vi "play_FXP_AFMss_LinearDistEst_singleAxis.vi"() -> ()   [LabVIEW 2017]
uses:
  fpga_VIs/fpga_subVIs_ssxy/fixed-point-ss/typeDefs/FXPControlParams_distEst.ctl
  fpga_fp_interface_lib/fpga_interface_types/boolean_indicators.ctl
  <vilib>/Analysis/Matrix/Datatypes/RealMatrix.ctl
  <vilib>/userdefined/High Color/nirio_resource_hc.ctl
  <vilib>/Utility/error.llb/DialogType.ctl
  <vilib>/Analysis/Matrix/Numeric/Conversions/Matrix To Array - RM.vi
  <vilib>/Utility/file.llb/Read Delimited Spreadsheet (DBL).vi
  <vilib>/FPGAPlugInAG/cRIO-9082/niLvFpga_Open_cRIO-9082.vi
  <vilib>/rvi/interface/common/dynamic/niFpgaDynamicAddResources.vi
  <vilib>/FPGAPlugInAG/Dynamic/niLvFpga_Reset_Dynamic.vi
  <vilib>/rvi/interface/common/niFpgaWaitOnOcc.vi
  <vilib>/Utility/error.llb/Error Cluster From Error Code.vi
  <vilib>/rvi/errors/niLvFpgaAdjustHostInterfaceError.vi
  <vilib>/FPGAPlugInAG/Dynamic/niLvFpga_Run_Dynamic.vi
  <vilib>/RVI Host/nirviSupport.llb/nirviErrorClusterFromErrorCode.vi
  fpga_fp_interface_lib/write_FP_data_to_fpga.vi
  fpga_fp_interface_lib/acquire_FXP_18-5_FIFO_1.vi
  <vilib>/Utility/file.llb/Write To Spreadsheet File (DBL).vi
  <vilib>/Analysis/Matrix/Numeric/Conversions/Array To Matrix - RA2.vi
  <vilib>/FPGAPlugInAG/Dynamic/niLvFpga_Close_Dynamic.vi
  <vilib>/rvi/interface/nirviOpenFPGA/nirviOpenFPGA.xnode
  FPGA Bitfiles/afmimagingcontro_FPGATargetSPARTA_FXPAFMssLinearDi_nzyJCj76J+U.lvbitx
  <vilib>/rvi/interface/nirviMethod/nirviMethod.xnode
  <vilib>/rvi/interface/nirviReadWriteControl/nirviReadWriteControl.xnode
  <vilib>/rvi/interface/nirviCloseFPGA/nirviCloseFPGA.xnode
  <vilib>/rvi/errors/niLvFpgaMergeErrorWithErrorCode.vi
  <vilib>/rvi/interface/Simulation/niFpgaSimulationCallBeginRW.vi
  <vilib>/rvi/interface/nirviMethod/StockFPGA_InlinedMethodWaitForSingleIRQ.vi
  <vilib>/FPGAPlugInAG/Dynamic/niLvFpga_WaitOnIrq_Dynamic.vi
  <vilib>/FPGAPlugInAG/Dynamic/niLvFpga_AcknowledgeIrq_Dynamic.vi
  <vilib>/FPGAPlugInAG/Dynamic/niLvFpga_ConfigureFifo_Dynamic.vi
  <vilib>/Analysis/Matrix/NI_Matrix.lvlib
  <vilib>/FPGAPlugInAG/Dynamic/niLvFpga_WriteFifo_Dynamic.vi
  labview/utils_lib/utils.lvlib
  NiFpgaLv.dll
panel:
  out "Array":dbl[](array[numeric])
  in  "sat_ws":T1
  in  "sat_ds":T1
  in  "N_sat":i32
  out "elements left":i32=1
  in  "N_hyst":i32
  in  "w_s":T1
  in  "r_s":T1
  in  "TF Order":i32
  in  "den":T1
  in  "num":T1
  in  "Tab Control":T2(tab)
  in  "traj_path":path=path "Z:/mpc-journal/step-exps/traj_data.csv"
  in  "TsTicks":i32=1600
  in  "umax":dbl=1.0 format="%#_13g"
  in  "ymax":dbl=4.0 format="%#_13g"
  in  "Iters":i32=25
  in  "SettleTicks":i32=10
  in  "dry_run":bool=TRUE
  in  "control_data_path":path=path "Z:/mpc-journal/step-exps/FXP_lin_Controls01.csv"
  in  "outputDataPath":path=path "Z:/mpc-journal/step-exps/expOut_multiAxis_tmp.csv"
  out "ControlParams":T3={"umax"=3.0, "Ns_obs/cntrl"=0, "ref_f_VEC"=[0.0, 0.0], "du_max"=0.0, "Nbar"=0.0}
  in  "ABORT":bool
  out "XY Graph":cluster{dbl[], "2D Data Out":dbl[]}[](graph)
  in  "read_file":bool=TRUE
  in  "All_matrix":T1
  in  "Ns_obs/cntrl":u8=21
  in  "yref":T1
  in  "du_max":dbl=1.0 format="%#_13g"
  out "AllMatrix":dbl[](array[numeric])
  out "ControlMatrices":T4
  out "result_data":T1
  out "boolean  indicators":T5
  out "error out":errorcluster
  out "Empty Elements Remaining":u32
  out "size(s)":i32[](array[numeric])
  out "u_k out":fxp<+/-,32,5>
  out "AllMatHS Length":i32
  # "NOTE: Ns is the number of states in the plant. The number of states in the \nobserver is Ns+1. Thus, for B, L, C, and A, we use NS+1. For K and Xss, we use Ns\nbecause the controller does not operate on the disturbance state, Xd."
  # "yk\nulin\ndu\nu_inv\nIpow\nX"
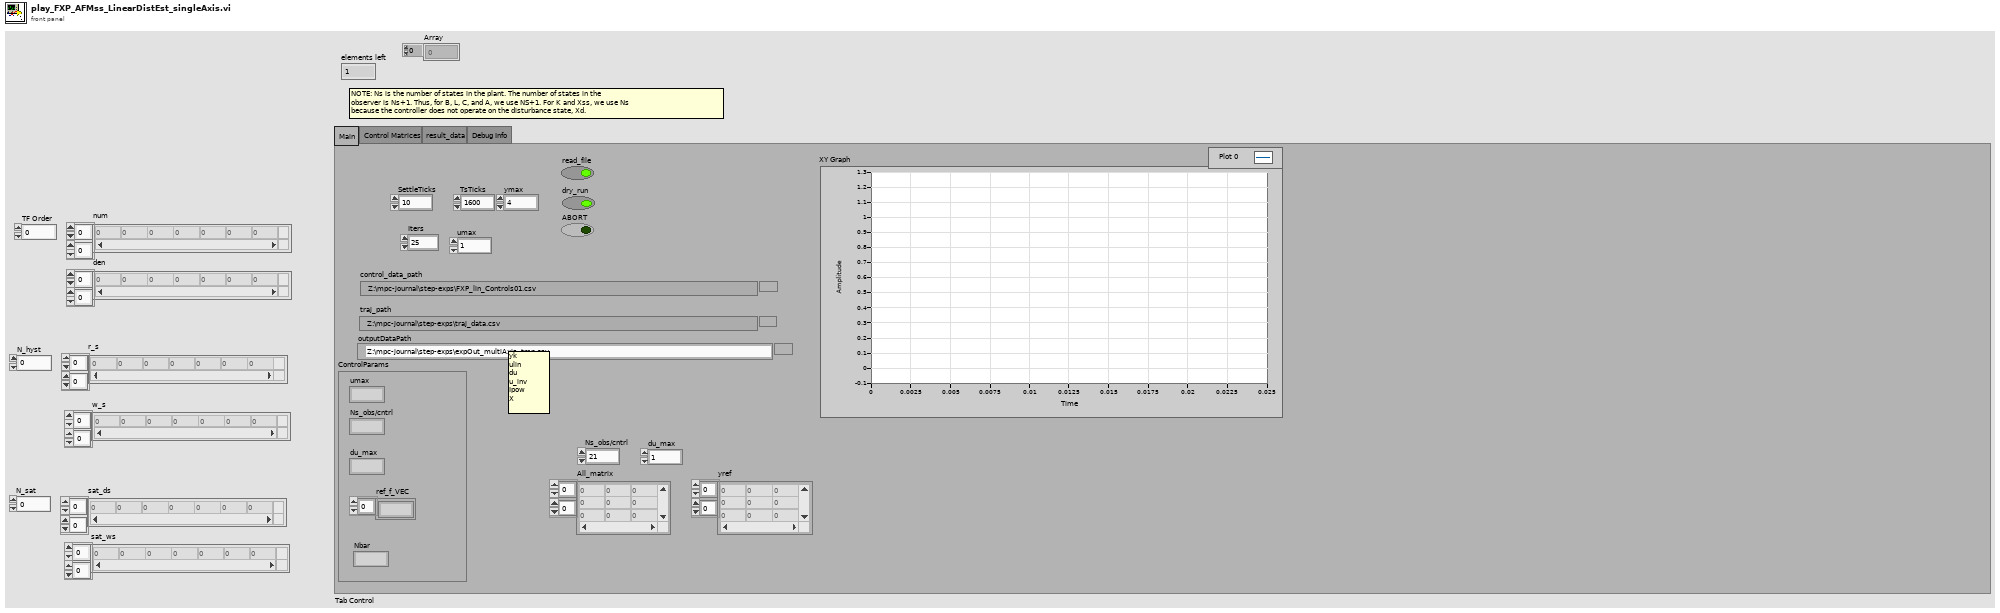
[diagram p1: front panel]
types:
  T1 = typedef "NI_Matrix.lvlib/RealMatrix.ctl" = dbl[][]
  T2 = enum32{"Main", "Control Matrices", "result_data", "Debug Info"}
  T3 = typedef "FXPControlParams_distEst.ctl" = cluster{"umax":fxp<+/-,18,5>, "Ns_obs/cntrl":u8, "ref_f_VEC":fxp<+/-,32,5>[], "du_max":fxp<+/-,18,5>, "Nbar":fxp<+/-,32,5>}
  T4 = cluster{"Az":fxp<+/-,32,4>[][], "Bz":dbl[][], "Lz":dbl[][], "Kz":dbl[][], "NxNu":dbl[][]}
  T5 = typedef "boolean_indicators.ctl" = cluster{"unstable-z-traj":bool, "input fifo time-out":bool, "logging fifo timeout":bool, "scanning finished":bool, "unstable-x-traj":bool, "unstable-y-traj":bool, "ABORT":bool, "All Measurements Done":bool, "fpga_finished":bool}
  T6 = typedef "nirio_resource_hc.ctl" = tag
  T7 = typedef "ObserverMatrices.ctl" = cluster{"Az":fxp<+/-,32,4>[][], "Bz":dbl[][], "Lz":dbl[][], "Kz":dbl[][], "NxNu":dbl[][]}
  T8 = cluster{"unstable-z-traj":bool, "input fifo time-out":bool, "logging fifo timeout":bool, "scanning finished":bool, "unstable-x-traj":bool, "unstable-y-traj":bool, "ABORT":bool, "All Measurements Done":bool, "fpga_finished":bool}
  T9 = typedef "DialogType.ctl" = u16
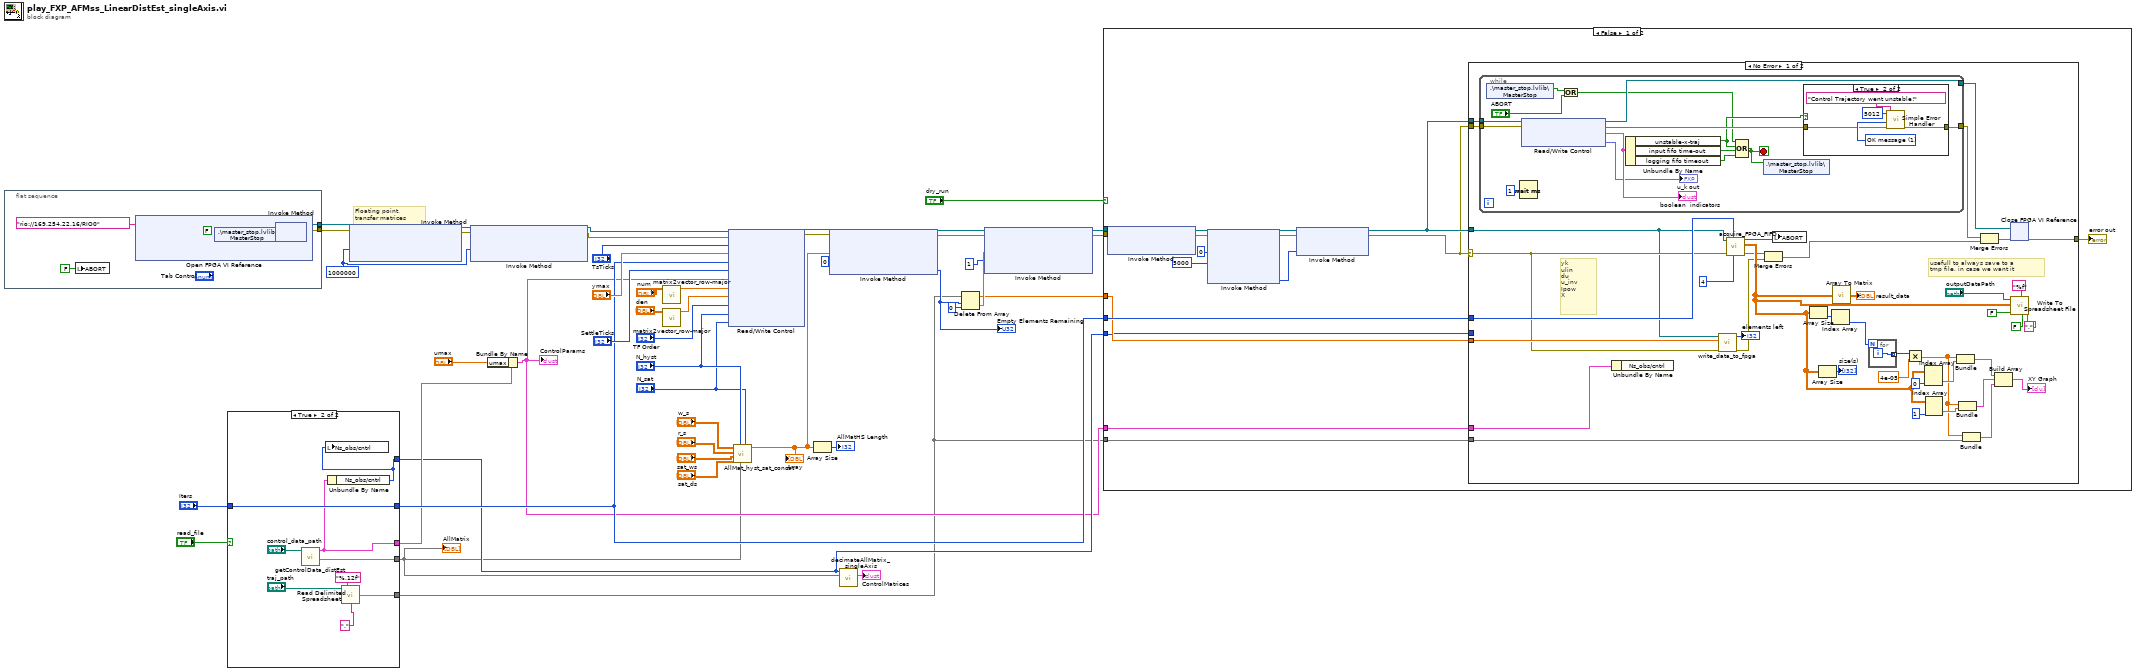
[diagram p0: block diagram]
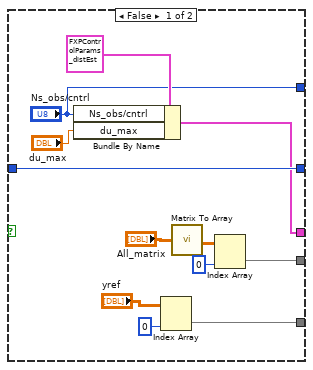
[diagram p2: hidden frame]
diagram:
  w12 = u32 1000000 ("Requested Depth")
  # "Floating point, \ntransfer matrices"
  n1 = flat-sequence {
    tunnel: [w53] -> w39
    tunnel: [w52] -> w38
    frame #0 {
      n2 = local write "ABORT"(FALSE) -> ()
      n3 = xnode "Open FPGA VI Reference"("resource name"=T6 "rio://169.254.22.16/RIO0") -> ("FPGA VI Reference Out"=w51:refnum<k20>, "error out"=w49:errorcluster)  [unwired: 1 in]
      n4 = shared-variable ".\\master_stop.lvlib\\MasterStop"(FALSE ("MasterStop"), error in=w49) -> (error out=w50:errorcluster)
      n5 = xnode "Invoke Method"("FPGA VI Reference In"=w51, "error in"=w50) -> ("FPGA VI Reference Out"=w53:refnum<k20>, "error out"=w52:errorcluster)
    }
  }
  n6 = case shown="True" "read_file" {
    tunnel: [w56 w68] -> w14
    tunnel: [w64 w74] -> w9
    tunnel: ["Ns_obs/cntrl" w67] -> w13
    tunnel: [w59 w71] -> w10
    tunnel: "Iters" -> [w62 w70]
    tunnel: [w62 w70] -> w15
    frame False {
      n7 = Bundle By Name(cluster=T3 {"umax"=3.0, "Ns_obs/cntrl"=0, "ref_f_VEC"=[0.0, 0.0], "du_max"=0.0, "Nbar"=0.0} ("ControlParams 2"), "Ns_obs/cntrl"="Ns_obs/cntrl", "du_max"="du_max") -> (w56:T3)
      n8 = Index Array(array="yref", index (col)=0 ("disabled index (col)")) -> (element=w59:dbl[])  [unwired: 1 in]
      n9 = call-poly <vilib>:"Matrix To Array.vi"("Real Matrix"="All_matrix") -> ("Real 2D Array"=w65:dbl[][])
      n10 = Index Array(array=w65, index (col)=0 ("disabled index (col)")) -> (element=w64:dbl[])  [unwired: 1 in]
    }
    frame True {
      n11 = call "getControlData_distEst.vi"("system matricec path"="control_data_path") -> ("AllMatrix"=w74:dbl[], "ControlParams"=w68:T3)  [unwired: 8 in, 1 out]
      n12 = Unbundle By Name(w68) -> ("Ns_obs/cntrl"=w67:u8)
      n13 = local write "Ns_obs/cntrl"(w67) -> ()
      n14 = call-poly <vilib>:"Read Delimited Spreadsheet.vi"("file path (dialog if empty)"="traj_path", "format (%.3f)"="%.12f", "delimiter (\\t)"="," ("format (%.3f)")) -> ("first row"=w71:dbl[])  [unwired: 7 in, 5 out]
    }
  }
  "AllMatrix" <- w9
  n15 = xnode "Invoke Method"("FPGA VI Reference In"=w39, "error in"=w38, "Requested Depth"=w12) -> ("FPGA VI Reference Out"=w37:refnum<k20>, "error out"=w36:errorcluster)  [unwired: 1 out]
  n16 = xnode "Invoke Method"("FPGA VI Reference In"=w37, "error in"=w36, "Requested Depth"=w12) -> ("FPGA VI Reference Out"=w34:refnum<k20>, "error out"=w35:errorcluster)  [unwired: 1 out]
  n17 = Bundle By Name(cluster=w14, "umax"="umax") -> (w11:T3)
  "ControlParams" <- w11
  n18 = call "matrix2vector_row-major.vi"("Matrix"="num") -> ("vector"=w28:dbl[])  [unwired: 10 in]
  n19 = call "matrix2vector_row-major.vi"("Matrix"="den") -> ("vector"=w27:dbl[])  [unwired: 10 in]
  n20 = xnode "Read/Write Control"("FPGA VI Reference In"=w34, "error in"=w35, "TsTicks"="TsTicks", "ymax"="ymax", "iters"=w15, "Settle Ticks"="SettleTicks", "ControlParamsMpc"=w11, "Num"=w28, "Den"=w27, "TF Order"="TF Order", "N_hyst"="N_hyst", "N_sat"="N_sat") -> ("FPGA VI Reference Out"=w43:refnum<k20>, "error out"=w42:errorcluster)
  n21 = call "AllMat_hyst_sat_concat.vi"("N_sat"="N_sat", "AllMatrix"=w9, "N_hyst"="N_hyst", "sat_ds"="sat_ds", "sat_ws"="sat_ws", "r_s"="r_s", "w_s"="w_s") -> ("Array"=w6:dbl[])  [unwired: 4 in]
  "Array" <- w6
  n22 = Array Size(array=w6) -> (size(s)=→"AllMatHS Length":i32)
  n23 = xnode "Invoke Method"("FPGA VI Reference In"=w43, "error in"=w42, "Data"=w6, "Timeout (ms)"=0) -> ("FPGA VI Reference Out"=w21:refnum<k20>, "error out"=w20:errorcluster, "Empty Elements Remaining"=w19:u32)
  "Empty Elements Remaining" <- w19
  n24 = call "decimateAllMatrix_singleAxis.vi"("AllMatrix"=w9, "NS_obs/cntrl"=w13) -> ("ControlMatrices"=→"ControlMatrices":T7)  [unwired: 8 in, 1 out]
  n25 = Delete From Array(array=w10, length=w19, index=0) -> (deleted portion=w25:dbl[], array with subset deleted=w17:dbl[])
  n26 = xnode "Invoke Method"("FPGA VI Reference In"=w21, "error in"=w20, "Data"=w25, "Timeout (ms)"=1) -> ("FPGA VI Reference Out"=w23:refnum<k20>, "error out"=w22:errorcluster)  [unwired: 1 out]
  n27 = case shown="False" "dry_run" {
    tunnel: w23 -> [w92 _]
    tunnel: w22 -> [w91 _]
    tunnel: w15 -> [w82 _]
    tunnel: w17 -> [w81 _]
    tunnel: w10 -> [w80 _]
    tunnel: w13 -> [w79 _]
    tunnel: w11 -> [w78 _]
    frame False {
      n28 = xnode "Invoke Method"("FPGA VI Reference In"=w92, "error in"=w91) -> ("FPGA VI Reference Out"=w85:refnum<k20>, "error out"=w86:errorcluster)  [unwired: 1 in]
      n29 = xnode "Invoke Method"("FPGA VI Reference In"=w85, "error in"=w86, "IRQ Number(s)"=0, "Timeout (ms)"=5000) -> ("FPGA VI Reference Out"=w89:refnum<k20>, "error out"=w90:errorcluster, "IRQ(s) Asserted"=w88:i32)  [unwired: 1 out]
      n30 = xnode "Invoke Method"("FPGA VI Reference In"=w89, "error in"=w90, "IRQ Number(s)"=w88) -> ("FPGA VI Reference Out"=w77:refnum<k20>, "error out"=w76:errorcluster)
      n31 = case shown="No Error" w76 {
        selector: w76 -> [w107 w154]
        tunnel: [w130 w154] -> w83
        tunnel: w77 -> [w129 _]
        tunnel: w76 -> [w128 _]
        tunnel: w82 -> [w125 _]
        tunnel: w77 -> [w97 _]
        tunnel: w81 -> [w108 _]
        tunnel: w80 -> [w101 _]
        tunnel: w79 -> [_ _]
        tunnel: w78 -> [w98 _]
        frame No Error {
          # "yk\nulin\ndu\nu_inv\nIpow\nX"
          # "usefull to always save to a \ntmp file, in case we want it"
          n32 = while {
            tunnel: w129 -> [w146]
            tunnel: w128 -> [w145]
            tunnel: [w143] -> w127
            tunnel: [w142] -> w126
            stop <- w141 stop-if-true
            n33 = shared-variable ".\\master_stop.lvlib\\MasterStop"() -> (w136:bool)  [unwired: 1 in, 1 out]
            n34 = Wait (ms)(milliseconds to wait=u32 1) -> ()  [unwired: 1 out]
            n35 = xnode "Read/Write Control"("FPGA VI Reference In"=w146, "error in"=w145) -> ("FPGA VI Reference Out"=w142:refnum<k20>, "error out"=w144:errorcluster, "boolean indicators"=w140:T8, "u_k"=→"u_k out":fxp<+/-,32,5>)
            "boolean  indicators" <- w140
            n36 = Or(x=w136, y="ABORT") -> (x .or. y?=w134:bool)
            n37 = Unbundle By Name(w140) -> ("unstable-x-traj"=w138:bool, "input fifo time-out"=w139:bool, "logging fifo timeout"=w137:bool)
            n38 = Compound Arithmetic op=OR(w134, w138, w139, w137) -> (w141:bool)
            n39 = shared-variable ".\\master_stop.lvlib\\MasterStop"(w141) -> ()  [unwired: 1 in, 1 out]
            n40 = case shown="True" w138 {
              tunnel: w144 -> [w148 w150]
              tunnel: [w148 w149] -> w143
              frame False {
              }
              frame True {
                w153 = T9 1 items=["no dialog", "OK message", "continue or stop message", "OK message + warnings", "continue/stop + warnings"] ("type of dialog (OK msg:1)")
                n41 = call <vilib>:"Simple Error Handler.vi"("error code (no error:0)"=5012, "error source (\" \")"="Control Trajectory went unstable!" ("error source (\" \")"), "type of dialog (OK msg:1)"=w153, "error in (no error)"=w150) -> ("error out"=w149:errorcluster)  [unwired: 1 in, 4 out]
              }
            }
          }
          n42 = Unbundle By Name(w98) -> ()  [unwired: 1 out]
          n43 = call-poly "write_data_to_fpga.vi"("error in"=w107, "all rows"=w108, "FPGA Interface"=w97) -> ("error out"=w104:errorcluster, "elements left"=→"elements left":i32)  [unwired: 7 in]
          n44 = call-poly "acquire_FPGA_FIFO.vi"("numChannels"=u8 4 ("y"), "Iters"=w125, "error in"=w107, "FPGA Interface"=w97) -> ("error out"=w106:errorcluster, "2D Data Out"=w122:dbl[][], "acquisition done"=w124:bool)  [unwired: 3 in, 2 out]
          n45 = Merge Errors(w106, w104) -> (w105:errorcluster)
          n46 = local write "ABORT"(w124) -> ()
          n47 = Array Size(array=w122) -> (size(s)=w118:i32[])
          n48 = Array Size(array=w122) -> (size(s)=→"size(s)":i32[])
          n49 = Index Array(array=w118) -> (element=w117:i32)  [unwired: 1 in]
          n50 = call-poly <vilib>:"Array To Matrix.vi"("Real 2D Array"=w122) -> ("Real Matrix"=→"result_data":T1)
          n51 = for {
            N: w117 -> [_]
            tunnel: [w132] -> w116 mode=indexing
            i -> [w132]
          }
          n52 = Multiply(x=w116, y=4e-05) -> (x*y=w102:dbl[])
          n53 = Index Array(array=w122, index (col)=0 ("disabled index (col)")) -> (element=w114:dbl[])  [unwired: 1 in]
          n54 = Index Array(array=w122, index (col)=1 ("index (row)")) -> (element=w113:dbl[])  [unwired: 1 in]
          n55 = Bundle(w102, "2D Data Out"=w114) -> (w95:cluster{dbl[], "2D Data Out":dbl[]})  [unwired: 1 in]
          n56 = Bundle(w102, "2D Data Out"=w113) -> (w94:cluster{dbl[], "2D Data Out":dbl[]})  [unwired: 1 in]
          n57 = Bundle(w102, "first row"=w101) -> (w93:cluster{dbl[], "first row":dbl[]})  [unwired: 1 in]
          n58 = Merge Errors(w127, w105) -> (w131:errorcluster)
          n59 = Build Array(w95, w94, w93) -> (→"XY Graph":cluster{dbl[], "first row":dbl[]}[])
          n60 = xnode "Close FPGA VI Reference"("FPGA VI Reference In"=w126, "error in"=w131) -> ("error out"=w130:errorcluster)
          n61 = call-poly <vilib>:"Write To Spreadsheet File.vi"("delimiter (\\t)"=",", "transpose? (no:F)"=FALSE, "format (%.3f)"="%f", "append to file? (new file:F)"=FALSE, "2D data"=w122, "file path (dialog if empty)"="outputDataPath") -> ()  [unwired: 2 in, 1 out]
        }
        frame Error {
        }
      }
      "error out" <- w83
    }
    frame True {
    }
  }
